vi "tdmsGenTool.vi"() -> ()   [LabVIEW 2026]
uses:
  <vilib>/platform/TimedLoop/XDataNode/XDataNode.xnode
  <vilib>/Platform/TimedLoop/XDataNode/nitl_modes.ctl
  <vilib>/Platform/TimedLoop/XDataNode/XDNodeRunTimeDep.lvlib
  <vilib>/Platform/TimedLoop/XDataNode/wakeup.ctl
  <vilib>/Platform/TimedLoop/XDataNode/timing_clust.ctl
  <vilib>/DAQmx/configure/timing.llb/DAQmx Timing (Sample Clock).vi
  <vilib>/DAQmx/create/channels.llb/DAQmx Create Channel (AI-Voltage-Basic).vi
  <vilib>/DAQmx/configure/task.llb/DAQmx Configure Logging (TDMS).vi
panel:
  in  "physical channels 2":tag
  in  "number of loops":i32=1
  in  "double?":bool
  in  "file format version (2.0)":enum16{"1.0", "2.0"}(ring)=enum."2.0"
  in  "create index file? (T)":bool=TRUE
  in  "byte order (2:little-endian)":T1(ring)
  in  "physical channels":tag[](array[tag])
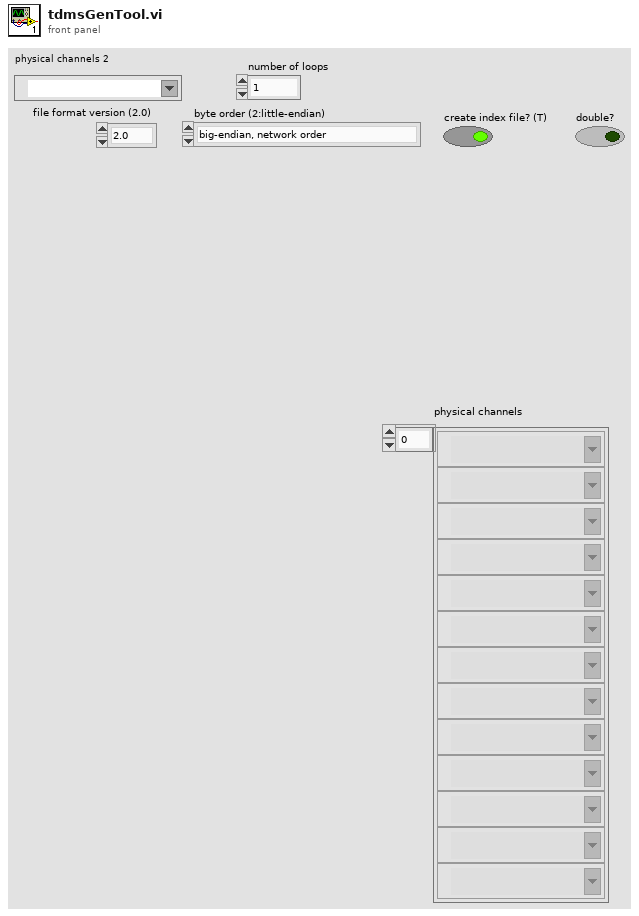
[diagram p1: front panel]
types:
  T1 = enum16{"big-endian, network order", "native, host order", "little-endian"}
  T2 = typedef "XDNodeRunTimeDep.lvlib/nitl_modes.ctl" = enum32{"No Change", "Process missed periods, maintain original phase", "Discard missed periods, maintain original phase", "Process missed periods, ignore original phase", "Discard missed periods, ignore original phase"}
  T3 = typedef "XDNodeRunTimeDep.lvlib/timing_clust.ctl" = cluster{"Expected End [f-1]":u64, "Actual End [f-1]":u64, "Finished Late? [f-1]":bool, "Expected End [i-1]":u64, "Actual End [i-1]":u64, "Finished Late? [i-1]":bool, "Expected Start [i]":u64, "Actual Start [i]":u64, "Expected Start [f]":u64, "Actual Start [f]":u64, "Source Name":string, "Structure Name":string, "Period":i64, "Deadline":i64, "Offset":i64, "Start":i64, "Priority":i32, "Timeout":i32, "Mode":T2, "Wakeup Reason":T4, "Error":errorcluster, "Source Type":string, "Secondary Source Type":string, "Global End Time":u64, "Global Start Time":u64, "Frame Duration":u64, "Iteration Duration":u64, "Assigned CPU":i32, "I/O Scan Engine Mode":u32}
  T4 = typedef "XDNodeRunTimeDep.lvlib/wakeup.ctl" = enum32{"Normal", "Aborted", "Asynchronous wakeup", "Timing source error", "Timed loop error", "Timeout"}
  T5 = enum16{"open", "open or create", "create or replace", "create", "open (read-only)"}
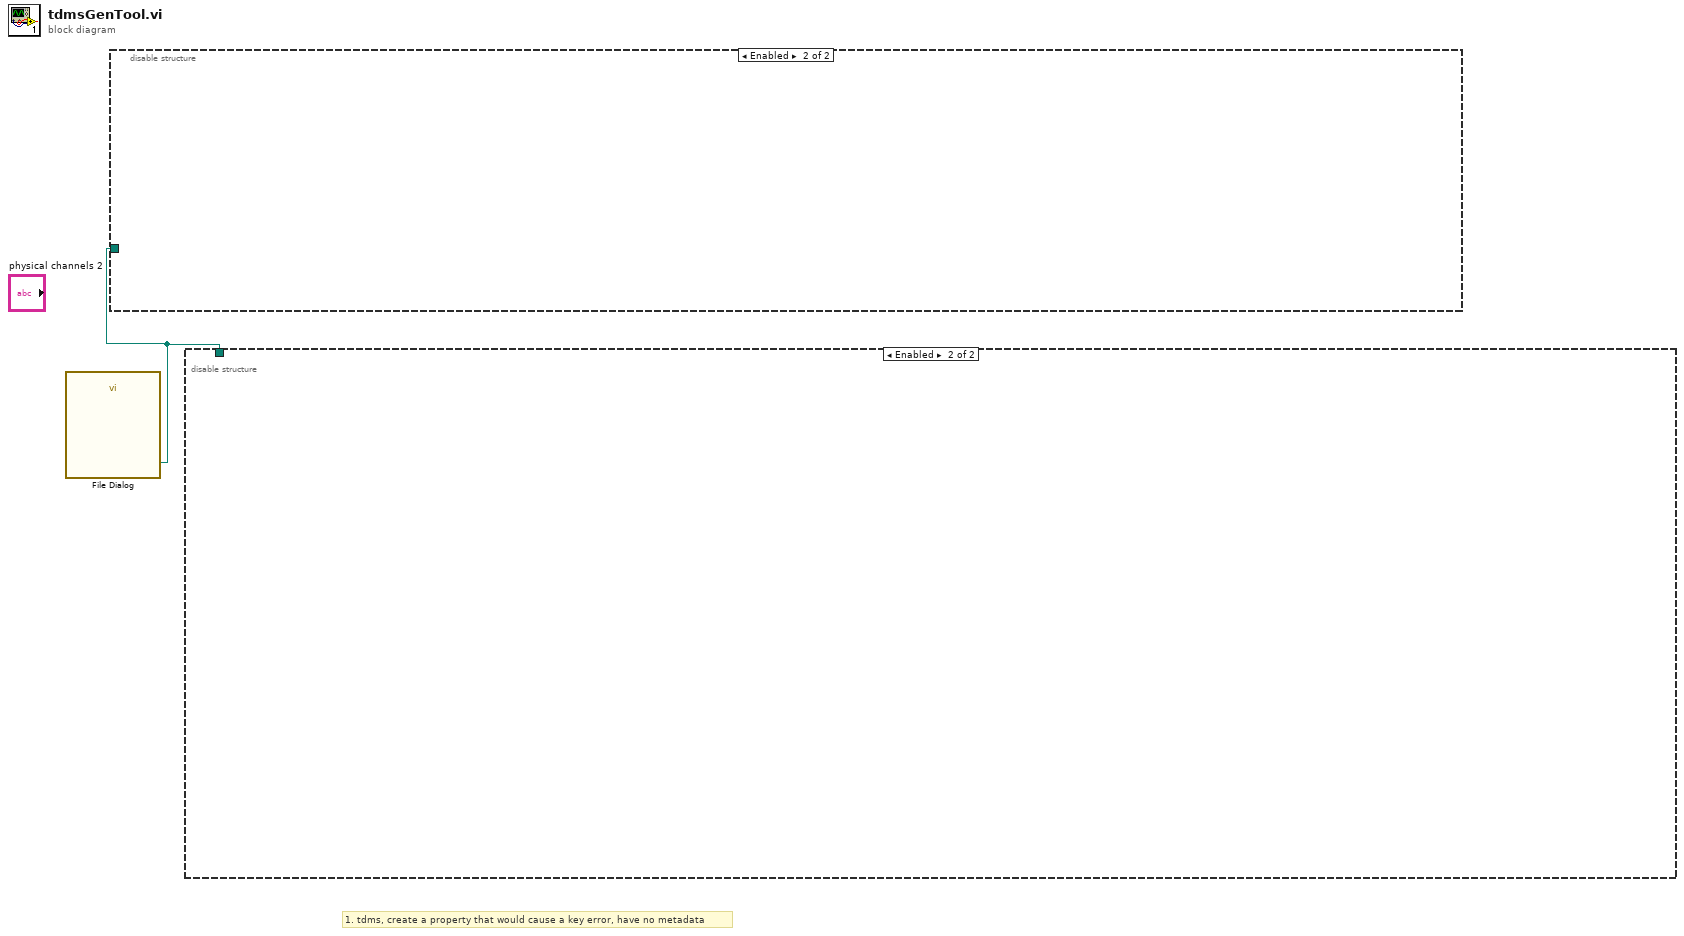
[diagram p0: block diagram]
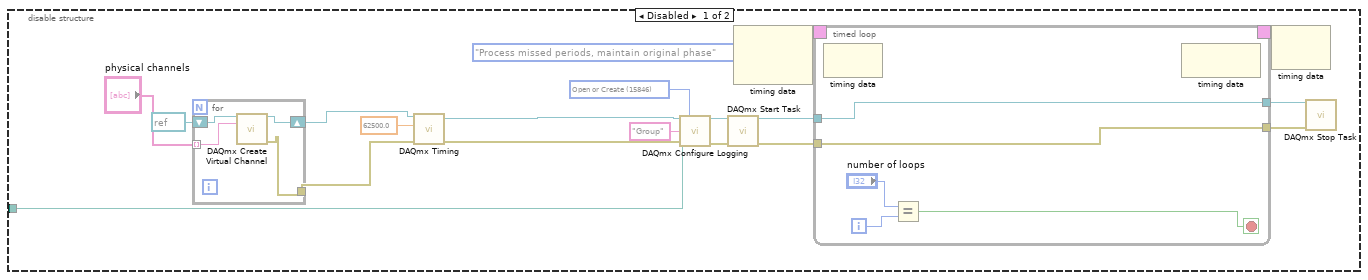
[diagram p2: hidden frame]
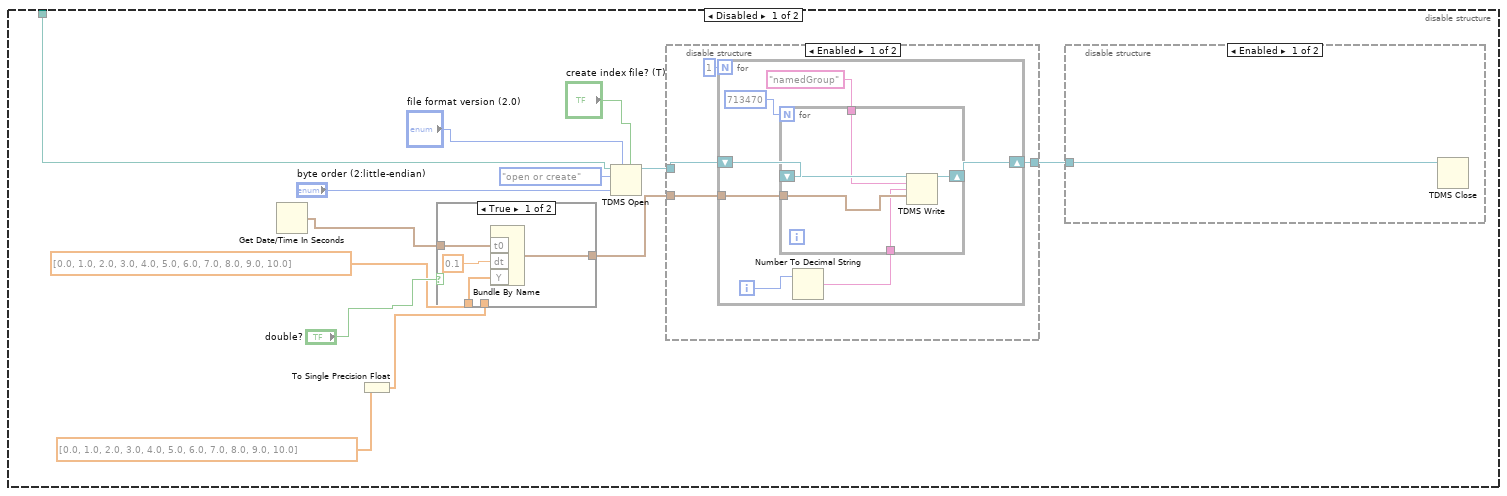
[diagram p3: hidden frame]
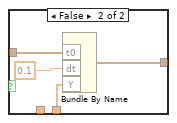
[diagram p6: hidden frame]
diagram:
  # "1. tdms, create a property that would cause a key error, have no metadata"
  n1 = call "File Dialog"() -> ("selected path"=w1:path)  [unwired: 12 in, 3 out]
  n2 = disable-structure shown="Enabled" {
    disable-tunnel: w1 -> [w6 _]
    frame Disabled {
      w17 = 15846 items=["Open"=10437, "Open or Create"=15846, "Create or Replace"=15847, "Create"=15848] ("operation")
      n3 = for {
        tunnel: [w23] -> w4
        tunnel: "physical channels" -> [w22] mode=indexing
        shift-right: [w24] -> w5
        shift-left: refnum<k21> refnum ("task out") -> [w21]
        n4 = call-poly <vilib>:"DAQmx Create Virtual Channel.vi"("task in"=w21, "physical channels"=w22) -> ("task out"=w24:refnum<k21>, "error out"=w23:errorcluster)  [unwired: 12 in]
      }
      n5 = call-poly <vilib>:"DAQmx Timing.vi"("task/channels in"=w5, "rate"=62500.0, "error in"=w4) -> ("task out"=w15:refnum<k21>, "error out"=w14:errorcluster)  [unwired: 11 in]
      n6 = call-poly <vilib>:"DAQmx Configure Logging.vi"("task/channels in"=w15, "operation"=w17, "file path"=w6, "group name"="Group", "error in"=w14) -> ("task out"=w13:refnum<k21>, "error out"=w12:errorcluster)  [unwired: 9 in]
      n7 = call <vilib>:"DAQmx Start Task.vi"("task/channels in"=w13, "error in"=w12) -> ("task out"=w11:refnum<k21>, "error out"=w10:errorcluster)  [unwired: 12 in]
      n8 = node-c288(nitl_modes."Process missed periods, maintain original phase" ("Mode")) -> (w20:T3)  [unwired: 1 in]
      n9 = timed-loop {
        tunnel: w11 -> [w27]
        tunnel: w10 -> [w26]
        timing: w20 -> [_]
        timing-out: [_] -> w19
        tunnel: [w27] -> w9
        tunnel: [w26] -> w8
        i -> [w29]
        stop <- w28 stop-if-true
        n10 = node-c288() -> ()  [unwired: 1 in, 1 out]
        n11 = Equal?(x="number of loops", y=w29) -> (x = y?=w28:bool)
        n12 = node-c288() -> ()  [unwired: 1 in, 1 out]
      }
      n13 = node-c288(w19) -> ()  [unwired: 1 out]
      n14 = call <vilib>:"DAQmx Stop Task.vi"("task/channels in"=w9, "error in"=w8) -> ()  [unwired: 12 in, 2 out]
    }
    frame Enabled {
    }
  }
  n15 = disable-structure shown="Enabled" {
    disable-tunnel: w1 -> [w46 _]
    frame Disabled {
      n16 = Get Date/Time In Seconds() -> (seconds since 1Jan1904=w39:timestamp)
      n17 = To Single Precision Float(number=dbl[] [0.0, 1.0, 2.0, 3.0, 4.0, 5.0, 6.0, 7.0, 8.0, 9.0, 10.0] ("Y")) -> (single precision float=w40:sgl[])
      n18 = case shown="True" "double?" {
        tunnel: w39 -> [w70 w74]
        tunnel: [w68 w72] -> w37
        tunnel: dbl[] [0.0, 1.0, 2.0, 3.0, 4.0, 5.0, 6.0, 7.0, 8.0, 9.0, 10.0] ("Y") -> [w67 _]
        tunnel: w40 -> [_ w71]
        frame True {
          n19 = Bundle By Name("t0"=w70, "dt"=0.1, "Y"=w67) -> (w68:waveform(dbl))  [unwired: 1 in]
        }
        frame False {
          n20 = Bundle By Name("t0"=w74, "dt"=0.1, "Y"=w71) -> (w72:waveform(sgl))  [unwired: 1 in]
        }
      }
      n21 = TDMS Open(5:"create index file? (T)", 7:"file format version (2.0)", 9:"byte order (2:little-endian)", 10:T5."open or create" ("operation (0:open)"), 11:w46) -> (3:w48:refnum<k34>)  [unwired: 2 in, 1 out]
      n22 = disable-structure shown="Enabled" {
        disable-tunnel: w48 -> [w52 w65]
        disable-tunnel: [w51 w65] -> w38
        disable-tunnel: w37 -> [w50 _]
        frame Enabled {
          n23 = for {
            N: 1 -> [_]
            tunnel: w50 -> [w55]
            shift-right: [w58] -> w51
            shift-left: w52 -> [w59]
            i -> [w54]
            n24 = Number To Decimal String(number=w54) -> (decimal integer string=w53:string)  [unwired: 1 in]
            n25 = for {
              N: 713470 -> [_]
              shift-right: [w63] -> w58
              shift-left: w59 -> [w64]
              tunnel: "namedGroup" ("group name in (Untitled)") -> [w62]
              tunnel: w55 -> [w61]
              tunnel: w53 -> [w60]
              n26 = TDMS Write(0:w64, 5:w62, 7:w60, 9:w61) -> (4:w63:refnum<k34>)  [unwired: 2 in, 3 out]
            }
          }
        }
        frame Disabled {
        }
      }
      n27 = disable-structure shown="Enabled" {
        disable-tunnel: w38 -> [w66 _]
        frame Enabled {
          n28 = TDMS Close(11:w66) -> ()  [unwired: 1 in, 2 out]
        }
        frame Disabled {
        }
      }
    }
    frame Enabled {
    }
  }
